vi "ReadFIFOConfig_HH.vi"(1 "error in (no error)":errorcluster) -> (0 "error out":errorcluster)   [LabVIEW 2009]
uses:
  SPCConfiguration.ctt
  FIFOSettings.ctt
  <vilib>/Utility/config.llb/NI_LVConfig.lvlib
panel:
  out "FIFO Settings":T1={"Measurement"={"Binning (ms)"=4719.0, "External Trigger Condition"=14979, "Stop Condition:"=0, "Stop Count"=0.0, "Buffer Size (Photons)"=30000, "No of Channels"=1, "Ext Latch Delay"=0}, "ADC"={"Binning (HH)"=0, "Dither Range"=0, "Count Increment"=0, "Mode"=1}, "SYNC"={"SYNC ZC Level (mV)"=-49.889763, "SYNC Freq Divider"=1, "SYNC Holdoff (ps)"=4.0, "SYNC Threshold (mV)"=-19.607843}, "TAC"={"TAC Range (ns)"=50.0, "TAC Gain"=0, "TAC Offset (%)"=0.0, "TAC Limit Low (%)"=0.0, "TAC Limit High (%)"=100.0}, "Ch 2"={"Ch2 ZC Level (mV)"=-43.137257, "Ch2 Holdoff (ps)"=67.76471, "Ch2 Threshold (mV)"=-49.889763}, "Ch 3"={"Ch3 ZC Level (mV)"=0.0, "Ch3 Holdoff (ps)"=4.0, "Ch3 Threshold (mV)"=200.0}, "Ch 4"={"Ch4 ZC Level (mV)"=0.0, "Ch4 Holdoff (ps)"=4.0, "Ch4 Threshold (mV)"=200.0}, "Ch1"={"Ch1 ZC Level (mV)"=0.0, "Ch1 Holdoff (ps)"=4.0, "Ch1 Threshold (mV)"=200.0}} {"Ch1"."Ch1 Threshold (mV)" min=0 max=1000 format="%.2f"; "Ch1"."Ch1 Holdoff (ps)" min=-99999 max=99999 format="%.2f"; "Ch1"."Ch1 ZC Level (mV)" min=0 max=40 format="%.2f"; "Ch 4"."Ch4 Threshold (mV)" min=0 max=1000 format="%.2f"; "Ch 4"."Ch4 Holdoff (ps)" min=-99999 max=99999 format="%.2f"; "Ch 4"."Ch4 ZC Level (mV)" min=0 max=40 format="%.2f"; "Ch 3"."Ch3 Threshold (mV)" min=0 max=1000 format="%.2f"; "Ch 3"."Ch3 Holdoff (ps)" min=-99999 max=99999 format="%.2f"; "Ch 3"."Ch3 ZC Level (mV)" min=0 max=40 format="%.2f"; "Ch 2"."Ch2 Threshold (mV)" min=-96 max=96 format="%.2f"; "Ch 2"."Ch2 Holdoff (ps)" min=4 max=80 format="%.2f"; "Ch 2"."Ch2 ZC Level (mV)" min=-500 max=80 format="%.2f"; "TAC"."TAC Limit High (%)" min=0 max=100 format="%.2f"; "TAC"."TAC Limit Low (%)" min=5 max=20 format="%.2f"; "TAC"."TAC Offset (%)" min=-96 max=96 format="%.2f"; "TAC"."TAC Gain" min=4 max=80; "TAC"."TAC Range (ns)" min=-500 max=80 format="%.2f"; "SYNC"."SYNC Threshold (mV)" min=5 max=20 format="%.2f"; "SYNC"."SYNC Holdoff (ps)" min=-96 max=96 format="%.2f"; "SYNC"."SYNC Freq Divider" items=["1", "2", "4", "8", "16"]; "SYNC"."SYNC ZC Level (mV)" min=-500 max=80 format="%.2f"; "ADC"."Mode" items=["T3"]; "ADC"."Binning (HH)" items=["1", "2", "4", "8", "16", "32", "64", "128", "256", "512", "1024"]; "ADC"."Count Increment" min=0 max=100; "ADC"."Dither Range" min=1 max=15 step=1; "Measurement"."Ext Latch Delay" min=0 max=255 step=1; "Measurement"."Stop Count" min=-500.0 max=-19.0 format="%.2f"; "Measurement"."Stop Condition:" items=["None", "Photon Count", "Time (s)"]; "Measurement"."External Trigger Condition" min=1 max=16 step=1; "Measurement"."No of Channels" max=14; "Measurement"."Binning (ms)" max=96 format="%.3f"}
  out "Storage Info":cluster{"Store Data":bool, "Destination:":path}
  out "SPC Configuration":T2={"SPC Initialization File"=path "SPC Labview Drivers/Important/spcm.ini", "Module Number"=0, "Operation Mode"=0, "Trigger Channel"="0"}
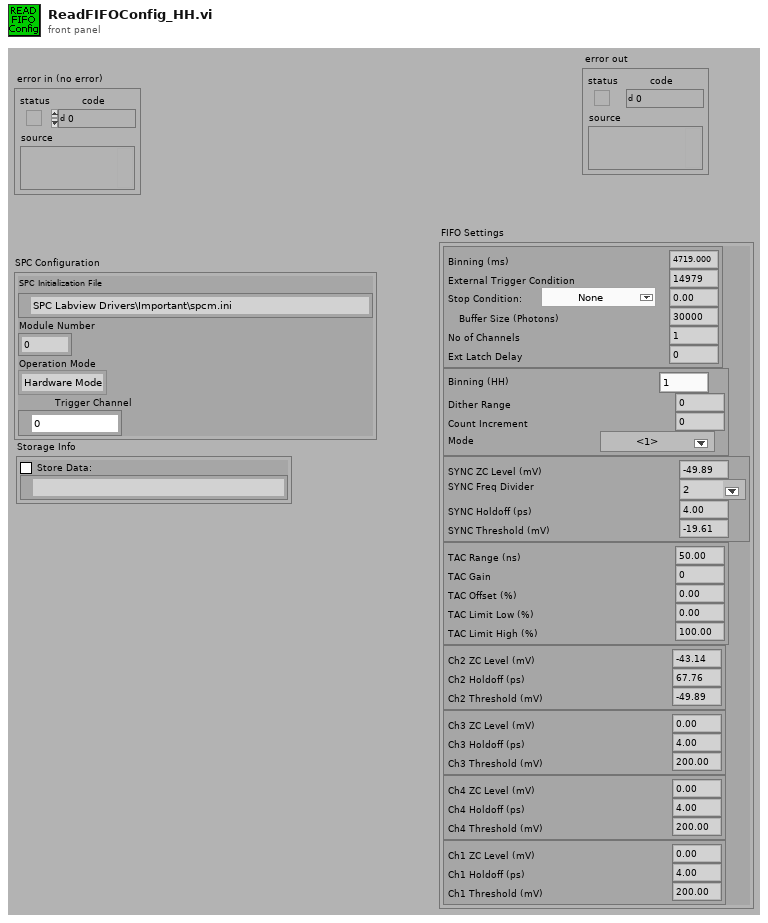
[diagram p1: front panel]
types:
  T1 = typedef "FIFOSettings.ctt" = cluster{"Measurement":cluster{"Binning (ms)":sgl, "External Trigger Condition":u16, "Stop Condition:":u16, "Stop Count":dbl, "Buffer Size (Photons)":u32, "No of Channels":u16, "Ext Latch Delay":i16}, "ADC":cluster{"Binning (HH)":i16, "Dither Range":i16, "Count Increment":i16, "Mode":u16}, "SYNC":cluster{"SYNC ZC Level (mV)":sgl, "SYNC Freq Divider":u16, "SYNC Holdoff (ps)":sgl, "SYNC Threshold (mV)":sgl}, "TAC":cluster{"TAC Range (ns)":sgl, "TAC Gain":i16, "TAC Offset (%)":sgl, "TAC Limit Low (%)":sgl, "TAC Limit High (%)":sgl}, "Ch 2":cluster{"Ch2 ZC Level (mV)":sgl, "Ch2 Holdoff (ps)":sgl, "Ch2 Threshold (mV)":sgl}, "Ch 3":cluster{"Ch3 ZC Level (mV)":sgl, "Ch3 Holdoff (ps)":sgl, "Ch3 Threshold (mV)":sgl}, "Ch 4":cluster{"Ch4 ZC Level (mV)":sgl, "Ch4 Holdoff (ps)":sgl, "Ch4 Threshold (mV)":sgl}, "Ch1":cluster{"Ch1 ZC Level (mV)":sgl, "Ch1 Holdoff (ps)":sgl, "Ch1 Threshold (mV)":sgl}}
  T2 = typedef "SPCConfiguration.ctt" = cluster{"SPC Initialization File":path, "Module Number":u16, "Operation Mode":u16, "Trigger Channel":tag}
  T3 = typedef "NI_LVConfig.lvlib/Config Data RefNum.ctl" = refnum<k1>
  T4 = cluster{"SPC Initialization File":path, "Module Number":u16, "Operation Mode":u16, "Trigger Channel":tag}
  T5 = cluster{"Measurement":cluster{"Binning (ms)":sgl, "External Trigger Condition":u16, "Stop Condition:":u16, "Stop Count":dbl, "Buffer Size (Photons)":u32, "No of Channels":u16, "Ext Latch Delay":i16}, "ADC":cluster{"Binning (HH)":i16, "Dither Range":i16, "Count Increment":i16, "Mode":u16}, "SYNC":cluster{"SYNC ZC Level (mV)":sgl, "SYNC Freq Divider":u16, "SYNC Holdoff (ps)":sgl, "SYNC Threshold (mV)":sgl}, "TAC":cluster{"TAC Range (ns)":sgl, "TAC Gain":i16, "TAC Offset (%)":sgl, "TAC Limit Low (%)":sgl, "TAC Limit High (%)":sgl}, "Ch 2":cluster{"Ch2 ZC Level (mV)":sgl, "Ch2 Holdoff (ps)":sgl, "Ch2 Threshold (mV)":sgl}, "Ch 3":cluster{"Ch3 ZC Level (mV)":sgl, "Ch3 Holdoff (ps)":sgl, "Ch3 Threshold (mV)":sgl}, "Ch 4":cluster{"Ch4 ZC Level (mV)":sgl, "Ch4 Holdoff (ps)":sgl, "Ch4 Threshold (mV)":sgl}, "Ch1":cluster{"Ch1 ZC Level (mV)":sgl, "Ch1 Holdoff (ps)":sgl, "Ch1 Threshold (mV)":sgl}}
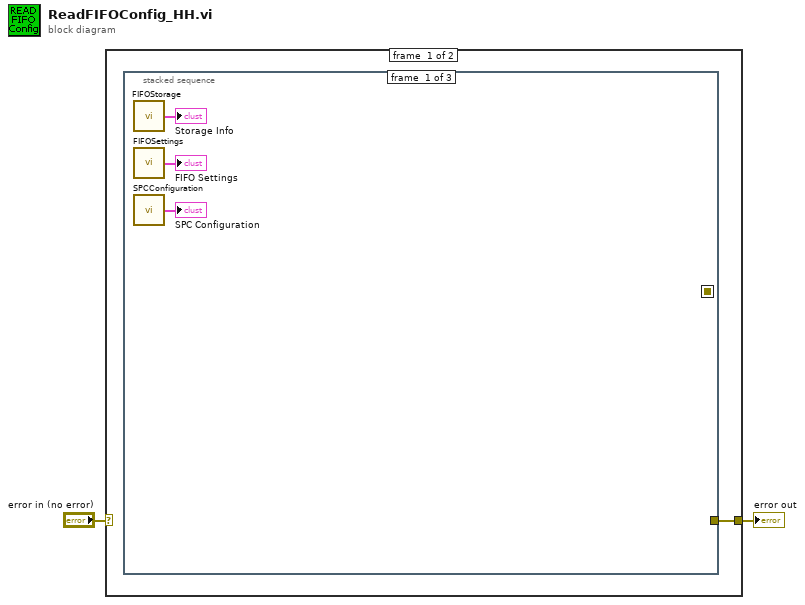
[diagram p0: block diagram]
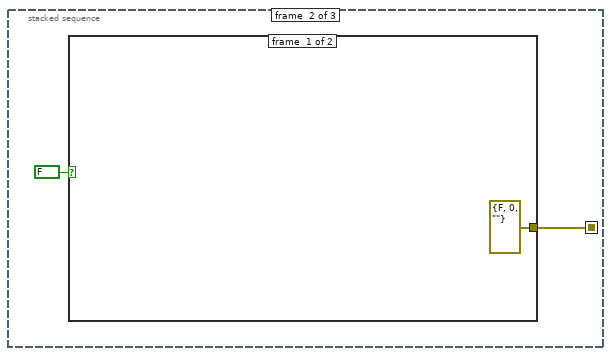
[diagram p2: hidden frame]
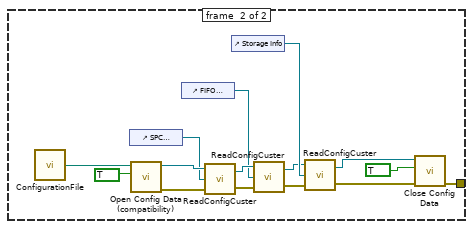
[diagram p3: hidden frame]
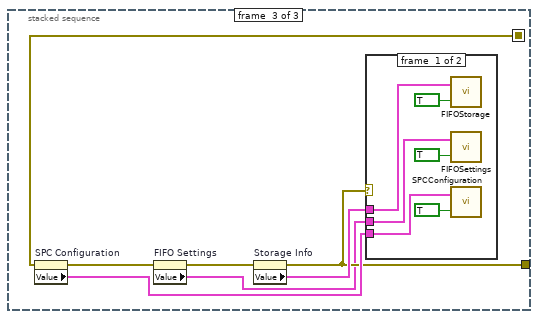
[diagram p4: hidden frame]
diagram:
  n1 = case shown="No Error" "error in (no error)" {
    selector: "error in (no error)" -> [_ w38]
    tunnel: [w3 w38] -> w1
    frame #0 {
      n2 = stacked-sequence {
        seq-local: [_ w8 _] -> [_ _ w29]
        tunnel: [_ _ w28] -> w3
        frame #0 {
          n3 = call "FIFOStorage.vi"() -> ("Storage Info (output)"=→"Storage Info":cluster{"Store Data":bool, "Destination:":path})  [unwired: 2 in]
          n4 = call "FIFOSettings.vi"() -> ("FIFO Settings(out)"=→"FIFO Settings":T1)  [unwired: 2 in]
          n5 = call "SPCConfiguration.vi"() -> ("SPC Configuration (output)"=→"SPC Configuration":T2)  [unwired: 2 in]
        }
        frame #1 {
          n6 = case shown="False" FALSE {
            tunnel: [errorcluster {"status"=FALSE, "code"=0, "source"=""} ("error out") w24] -> w8
            frame #0 {
            }
            frame #1 {
              n7 = call "ConfigurationFile.vi"() -> ("Configuration File (output)"=w11:path)  [unwired: 2 in]
              n8 = control-ref of="SPC Configuration"() -> (w21:refnum<vi>)
              n9 = call <vilib>:"Open Config Data (compatibility).vi"("create file if necessary (T)"=TRUE ("create file if necessary? (T)"), "configuration file path"=w11) -> ("error out"=w20:errorcluster, "refnum"=w22:T3)  [unwired: 7 in, 1 out]
              n10 = control-ref of="FIFO Settings"() -> (w10:refnum<vi>)
              n11 = call "ReadConfigCuster.vi"("error in (no error)"=w20, "Ctrl Reference"=w21, "ConfigFile (input)"=w22) -> ("error out"=w13:errorcluster, "ConfigFile (output)"=w14:T3)
              n12 = control-ref of="Storage Info"() -> (w19:refnum<vi>)
              n13 = call "ReadConfigCuster.vi"("error in (no error)"=w13, "Ctrl Reference"=w10, "ConfigFile (input)"=w14) -> ("error out"=w12:errorcluster, "ConfigFile (output)"=w15:T3)
              n14 = call "ReadConfigCuster.vi"("error in (no error)"=w12, "Ctrl Reference"=w19, "ConfigFile (input)"=w15) -> ("error out"=w17:errorcluster, "ConfigFile (output)"=w16:T3)
              n15 = call "Close Config Data.vi"("error in (no error)"=w17, "write configuration file? (T)"=TRUE ("write configuration file? (F)"), "refnum"=w16) -> ("error out"=w24:errorcluster)  [unwired: 8 in]
            }
          }
        }
        frame #2 {
          n16 = property on="SPC Configuration" class="Clust (strict)"(error in=w29) -> (error out=w26:errorcluster, "Value"=w30:T4)  [unwired: 1 in, 1 out]
          n17 = property on="FIFO Settings" class="Cluster (strikt)"(error in=w26) -> (error out=w25:errorcluster, "Value"=w27:T5)  [unwired: 1 in, 1 out]
          n18 = property on="Storage Info" class="Cluster (strict)"(error in=w25) -> (error out=w28:errorcluster, "Value"=w31:cluster{"Store Data":bool, "Destination:":path})  [unwired: 1 in, 1 out]
          n19 = case shown="No Error" w28 {
            tunnel: w31 -> [w35 _]
            tunnel: w30 -> [w34 _]
            tunnel: w27 -> [w33 _]
            frame #0 {
              n20 = call "FIFOStorage.vi"("Set/Get"=TRUE ("Set"), "Storage Info (input)"=w35) -> ()  [unwired: 1 out]
              n21 = call "FIFOSettings.vi"("Set/Get"=TRUE ("Set"), "FIFO Settings(in)"=w33) -> ()  [unwired: 1 out]
              n22 = call "SPCConfiguration.vi"("Set/Get"=TRUE ("Set"), "SPC Configuration (input)"=w34) -> ()  [unwired: 1 out]
            }
            frame #1 {
            }
          }
        }
      }
    }
    frame #1 {
    }
  }
  "error out" <- w1
